vi "Serviceman.vi"() -> ()   [LabVIEW 2023]
uses:
  <vilib>/Utility/file.llb/Read Delimited Spreadsheet (string).vi
  <vilib>/Utility/file.llb/Write Delimited Spreadsheet (string).vi
panel:
  in  "Tab Control":T1(tab)=enum."Register_page"
  in  "register_btn":bool
  in  "login_btn":bool
  in  "password_login":string
  in  "username_login":string
  in  "home_btn":bool
  in  "back_to_login_btn":bool
  out "rgstr_status":string
  in  "email_address_rgstr":string
  in  "last_name_rgstr":string
  in  "first_name_rgstr":string
  in  "register_btn_rgstr":bool
  in  "password_rgstr":string
  in  "username_rgstr":string
  in  "logout_btn":bool
  # "Login"
  # "Username:"
  # "Password:"
  # "or Register"
  # "Registration"
  # "First Name:"
  # "Last Name:"
  # "Email Address:"
  # "Username:"
  # "Password:"
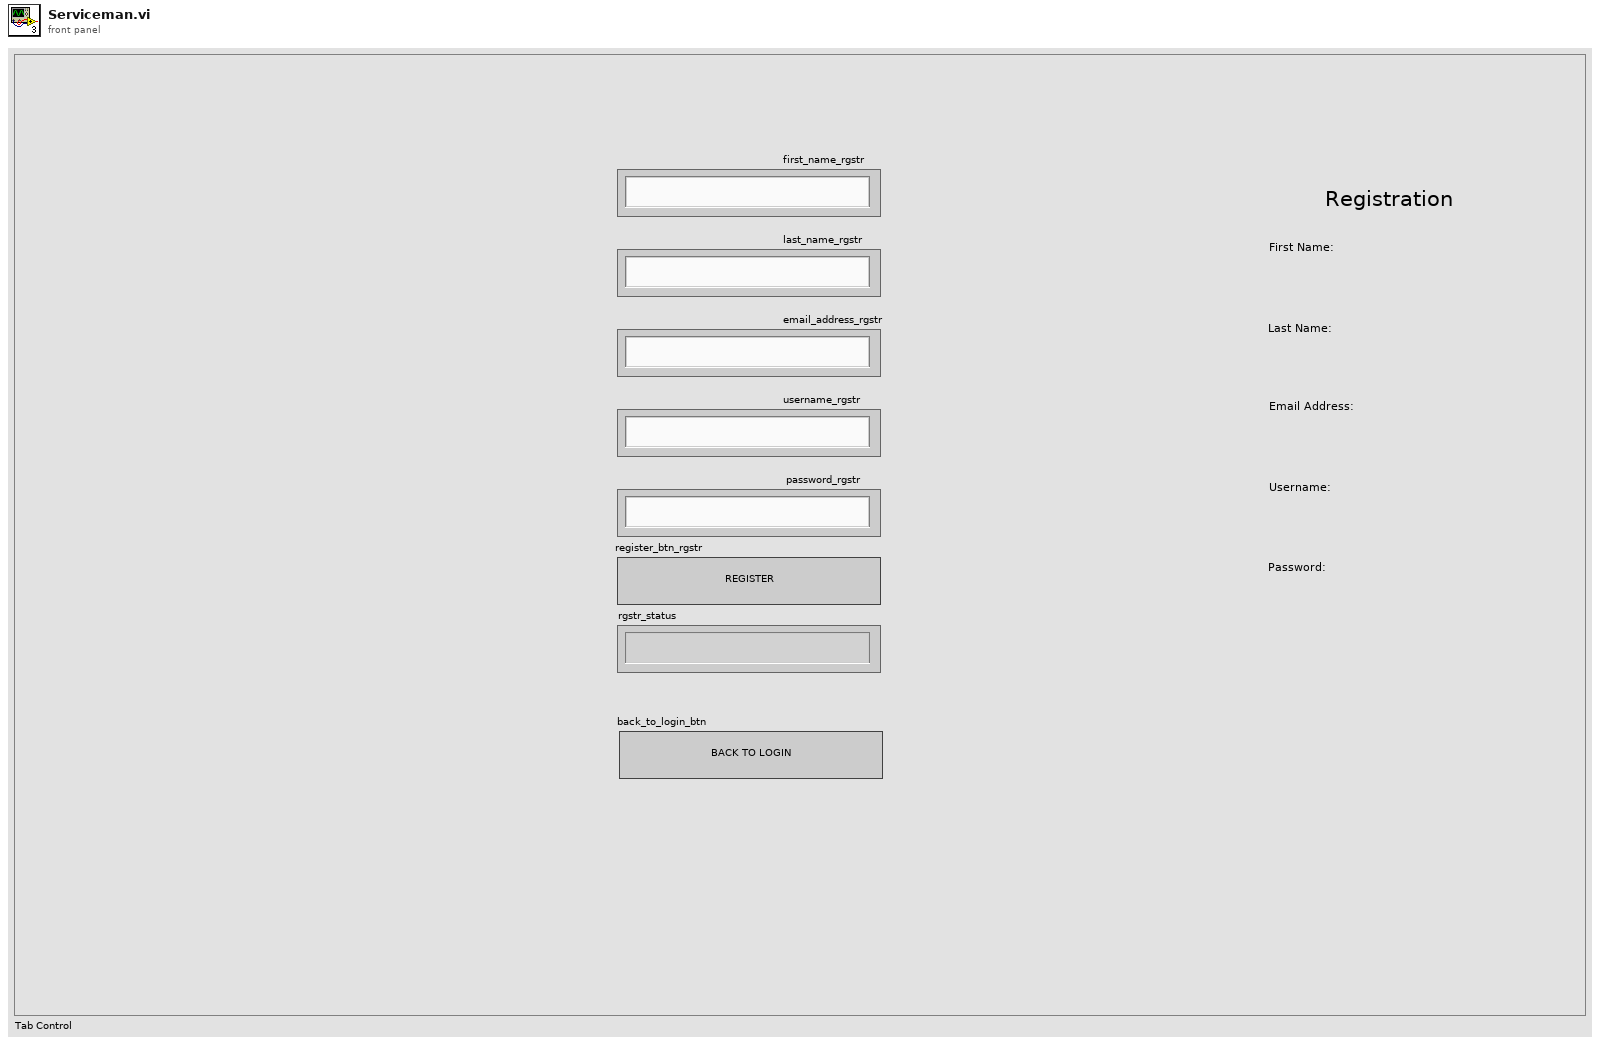
[diagram p1: front panel]
types:
  T1 = enum32{"Login_page", "Register_page", "Serviceman_page"}
  T2 = cluster{"Some":bool, "Tab Control":enum32{"Login_page", "Register_page", "Serviceman_page"}, "Probe":i32}
  T3 = enum16{"open", "replace", "create", "open or create", "replace or create", "replace or create with confirmation"}
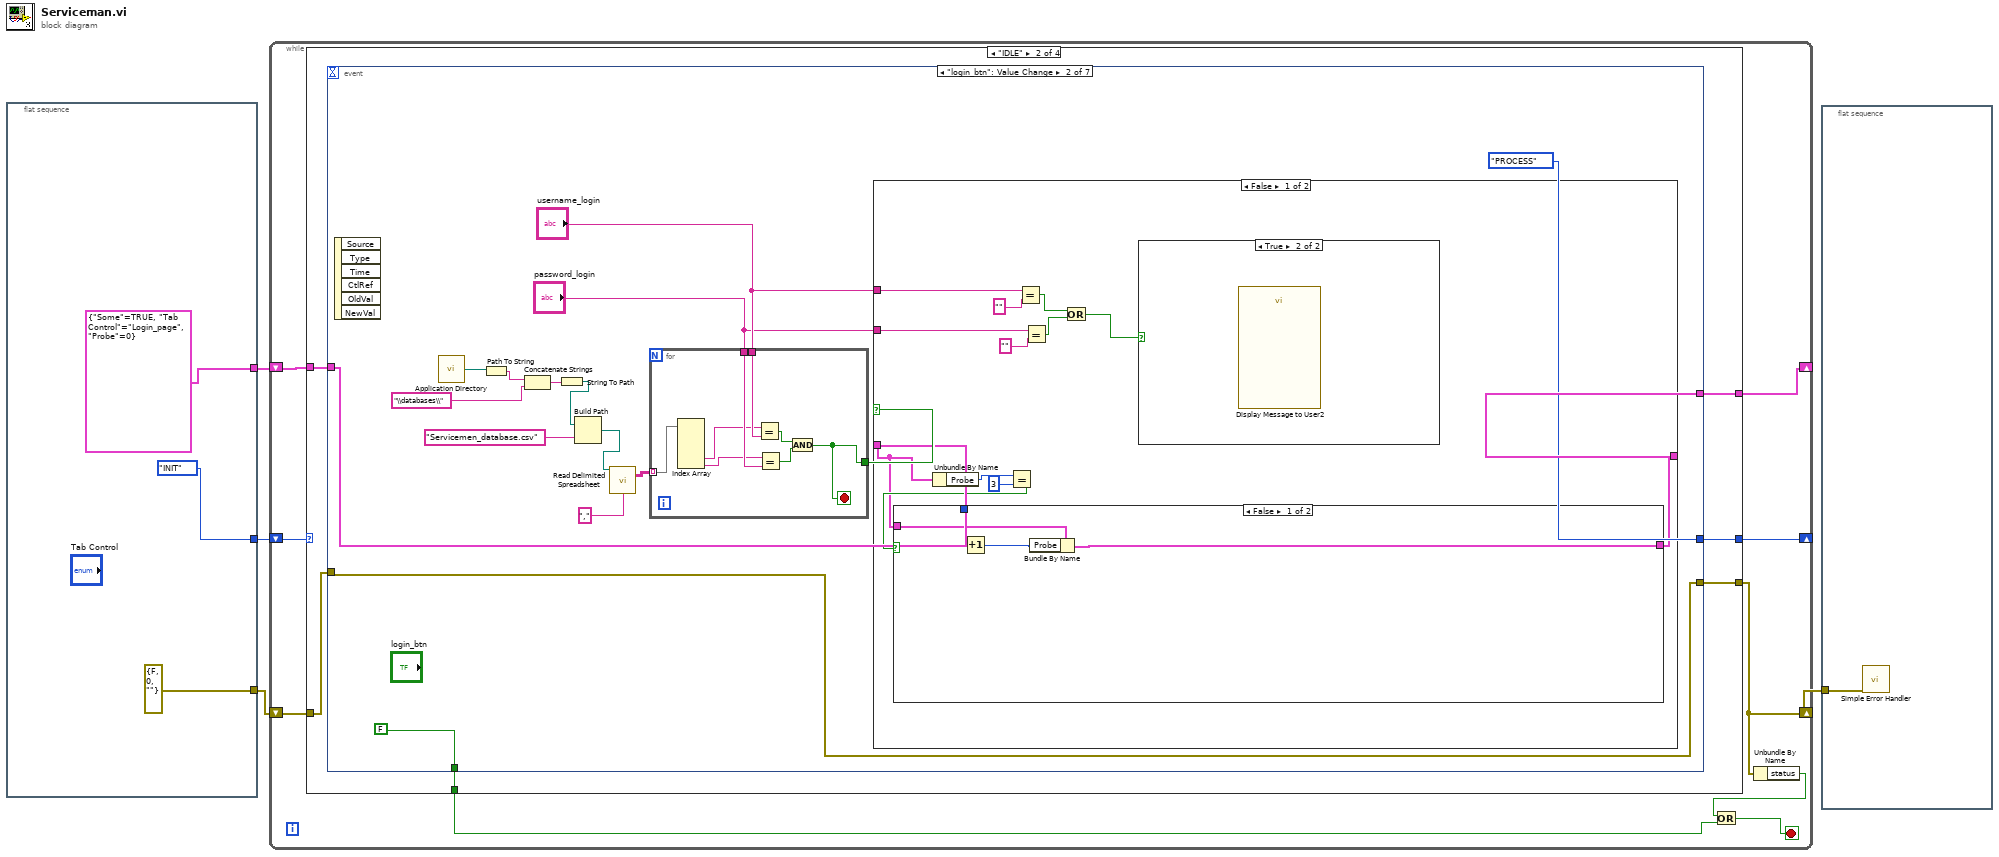
[diagram p0: block diagram]
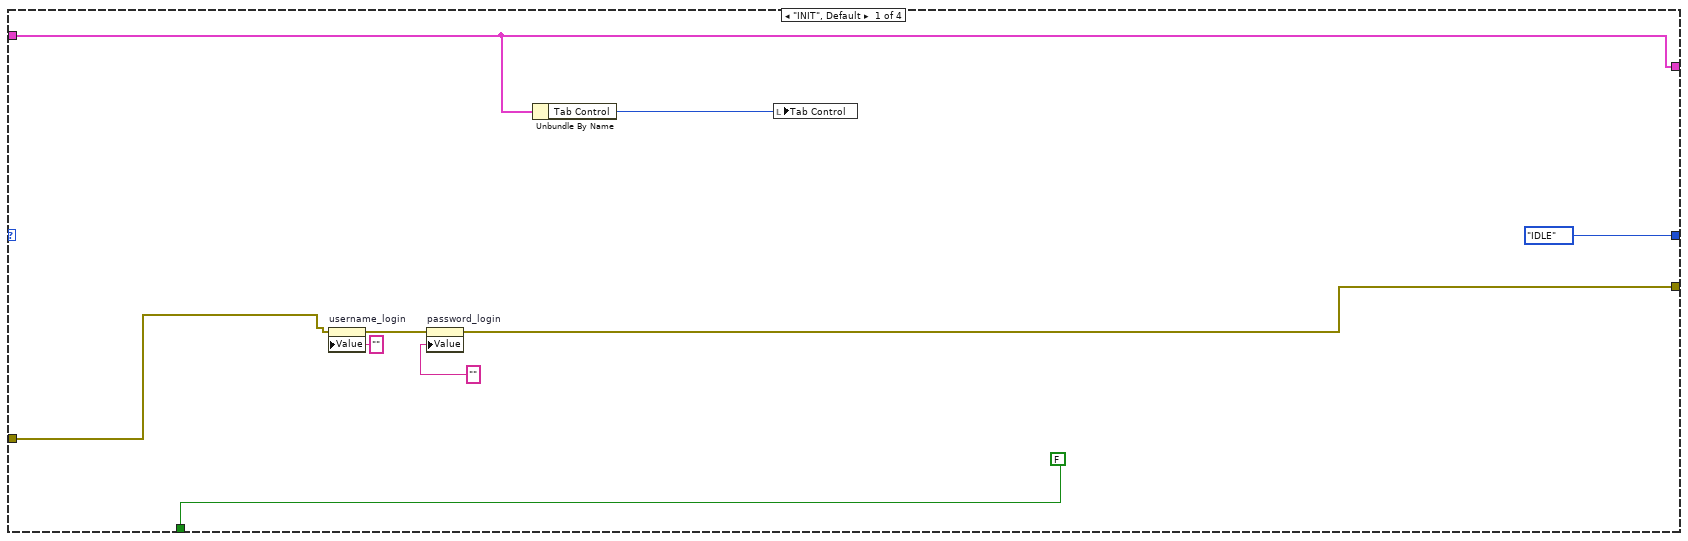
[diagram p2: hidden frame]
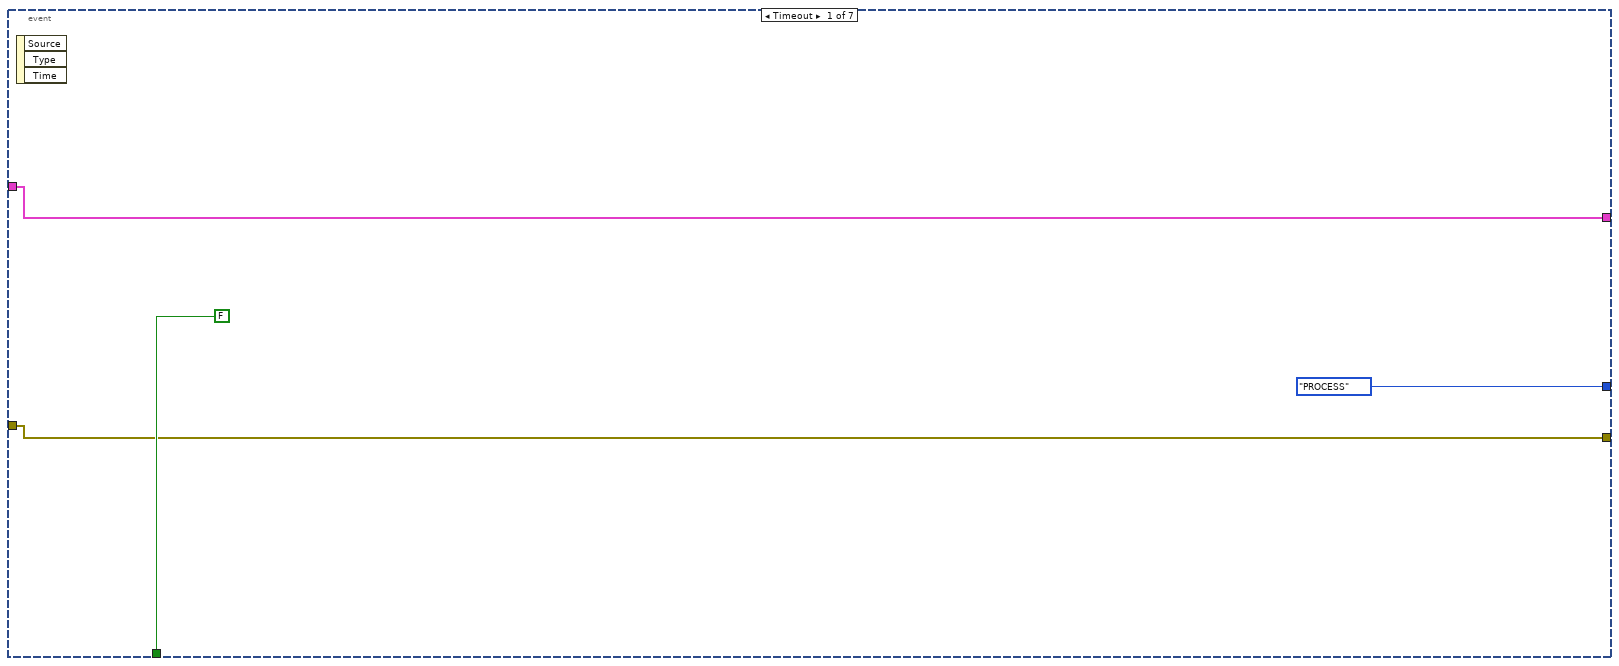
[diagram p3: hidden frame]
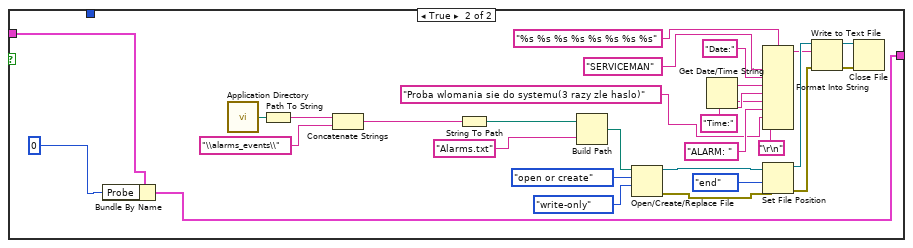
[diagram p4: hidden frame]
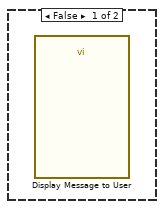
[diagram p5: hidden frame]
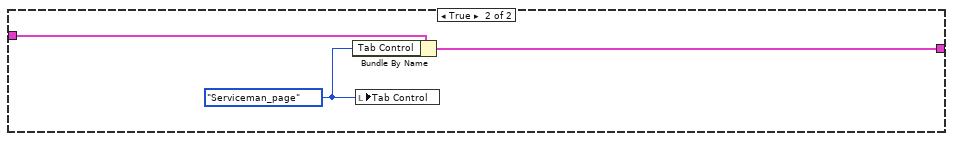
[diagram p6: hidden frame]
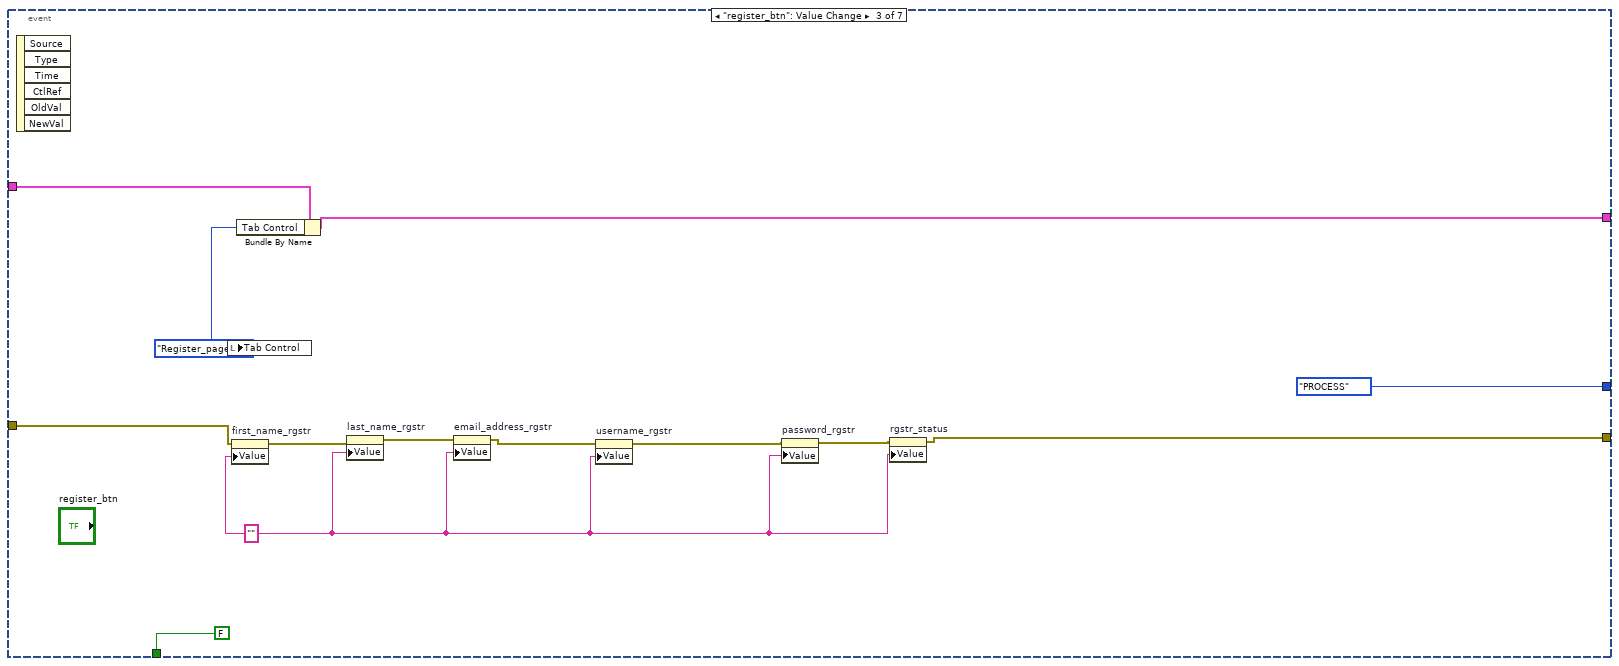
[diagram p7: hidden frame]
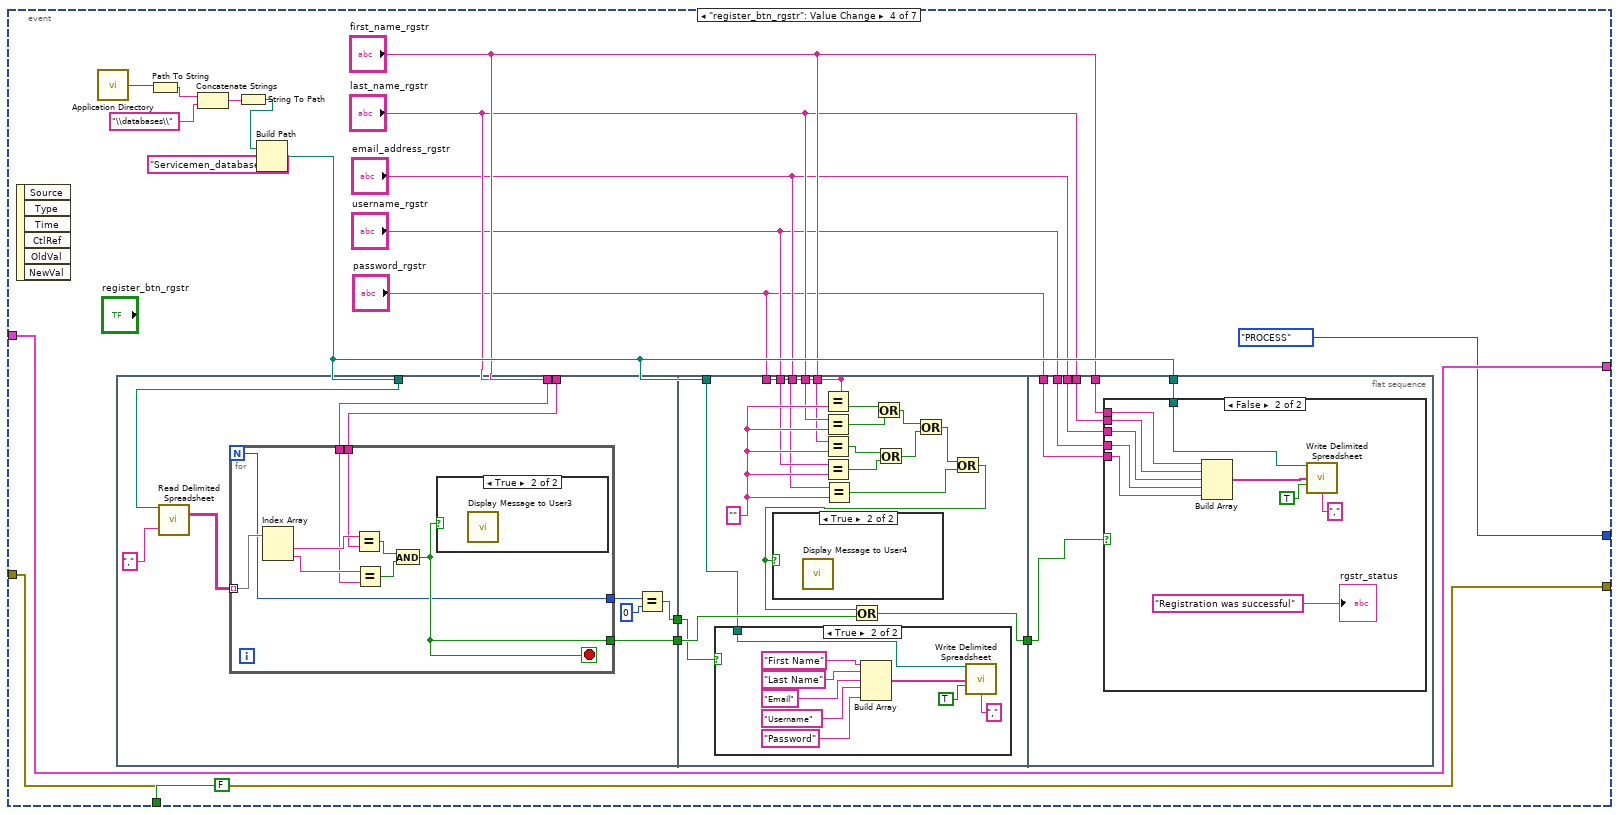
[diagram p8: hidden frame]
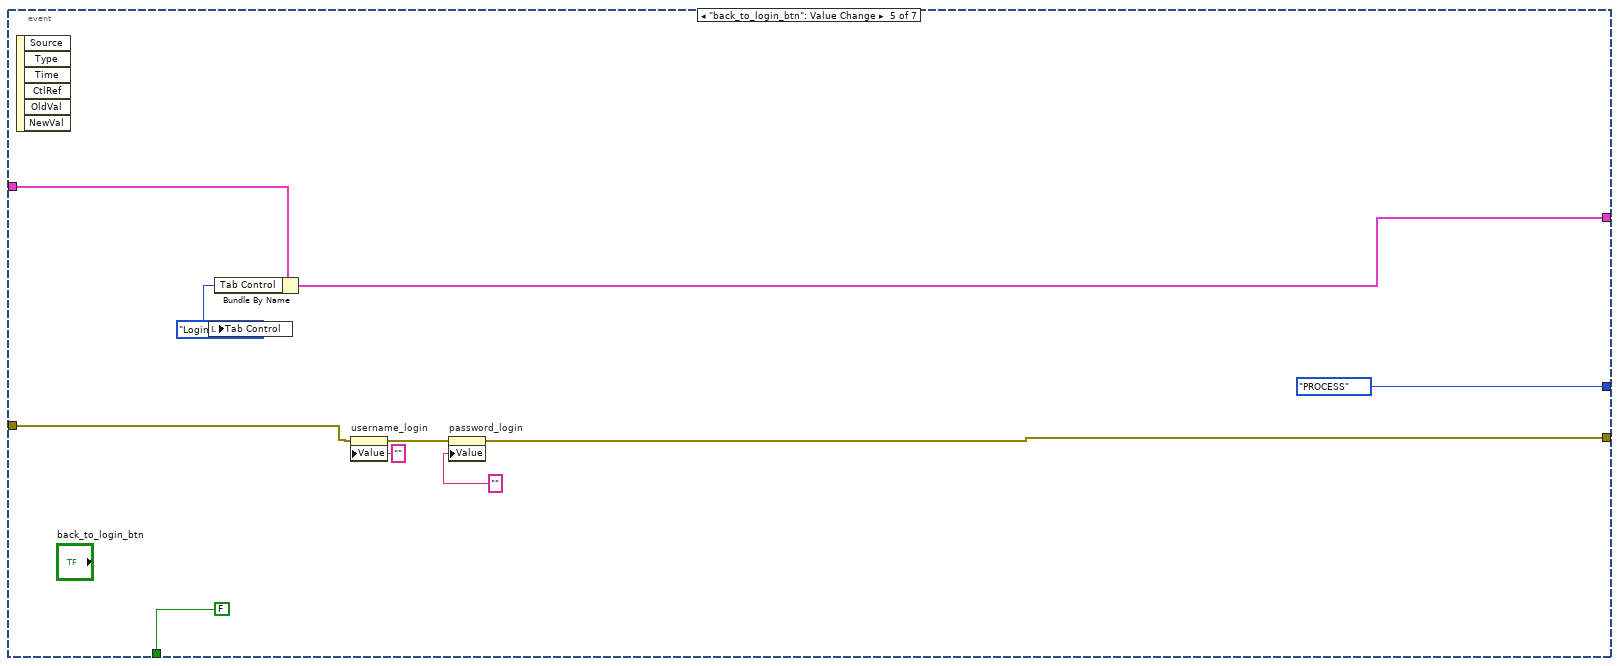
[diagram p13: hidden frame]
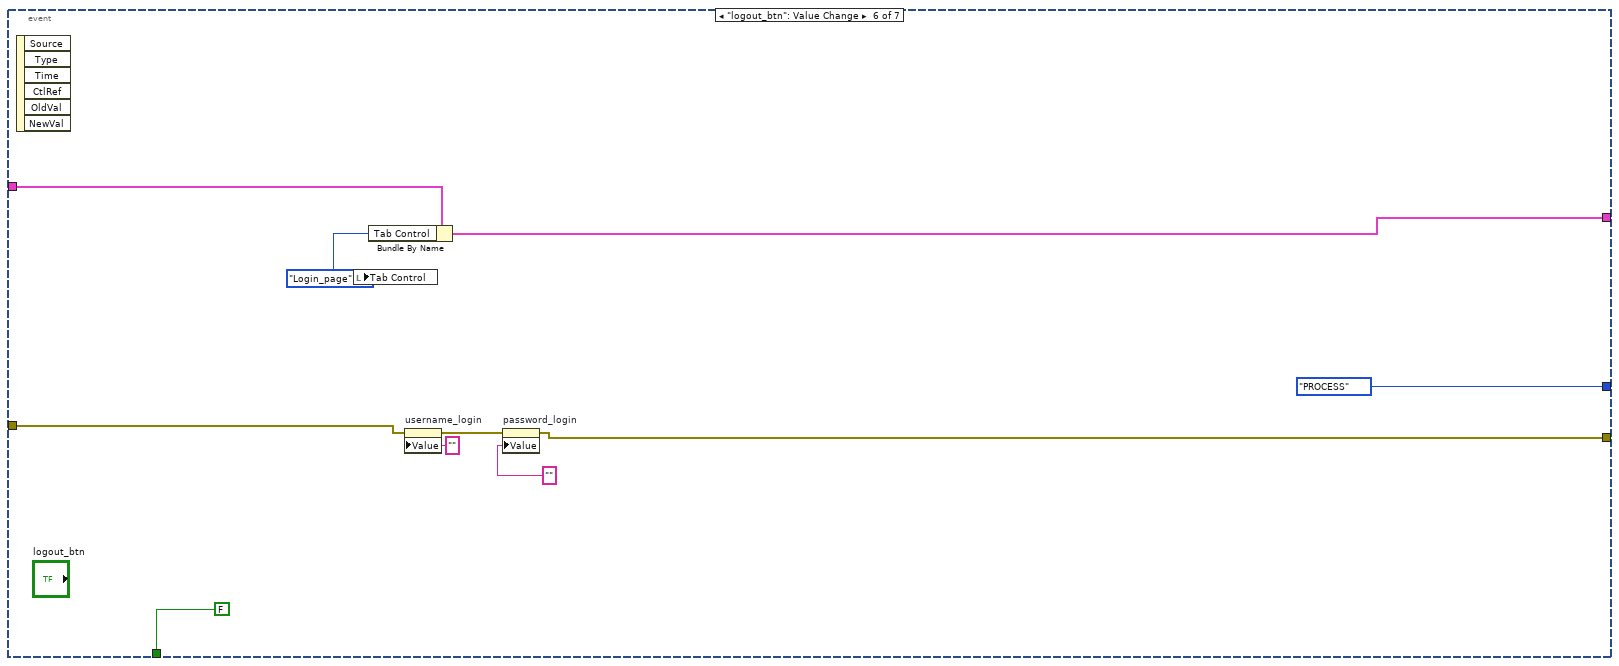
[diagram p14: hidden frame]
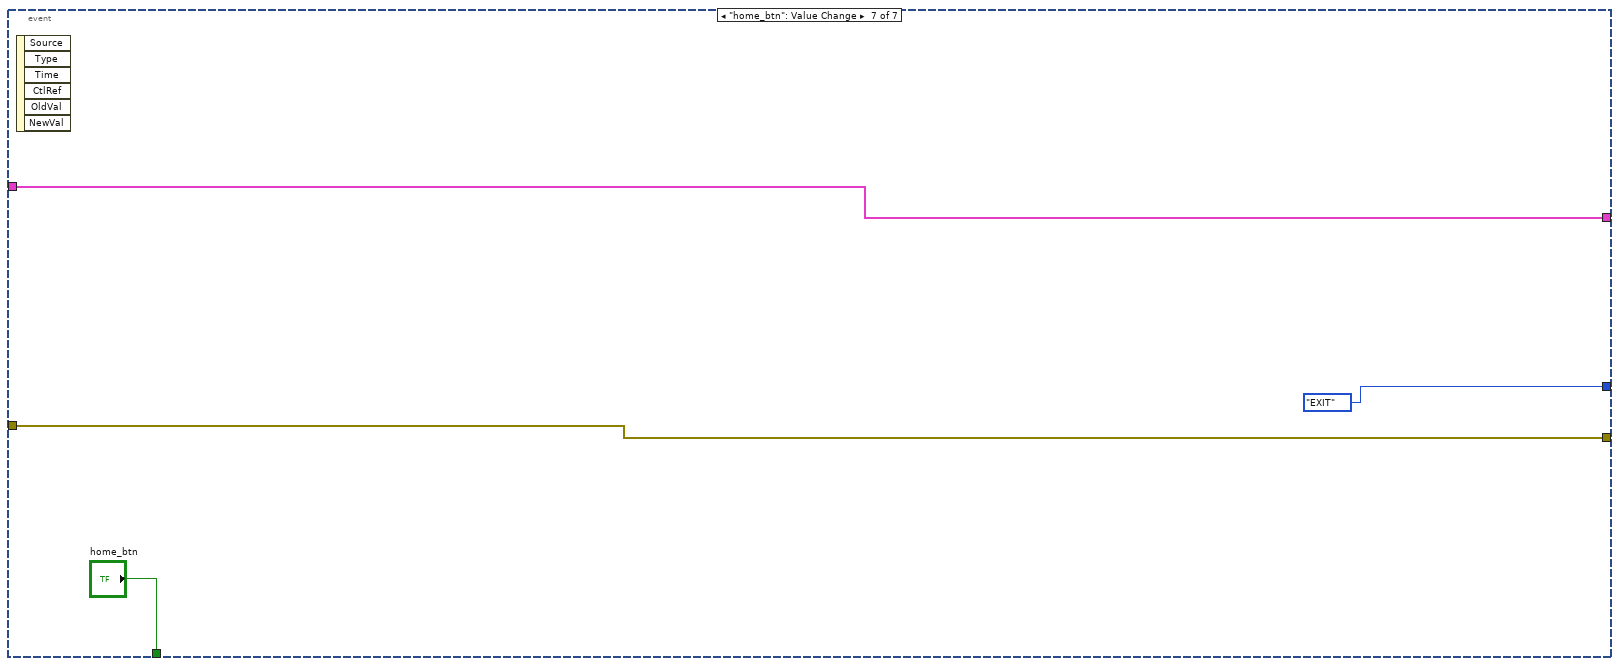
[diagram p15: hidden frame]
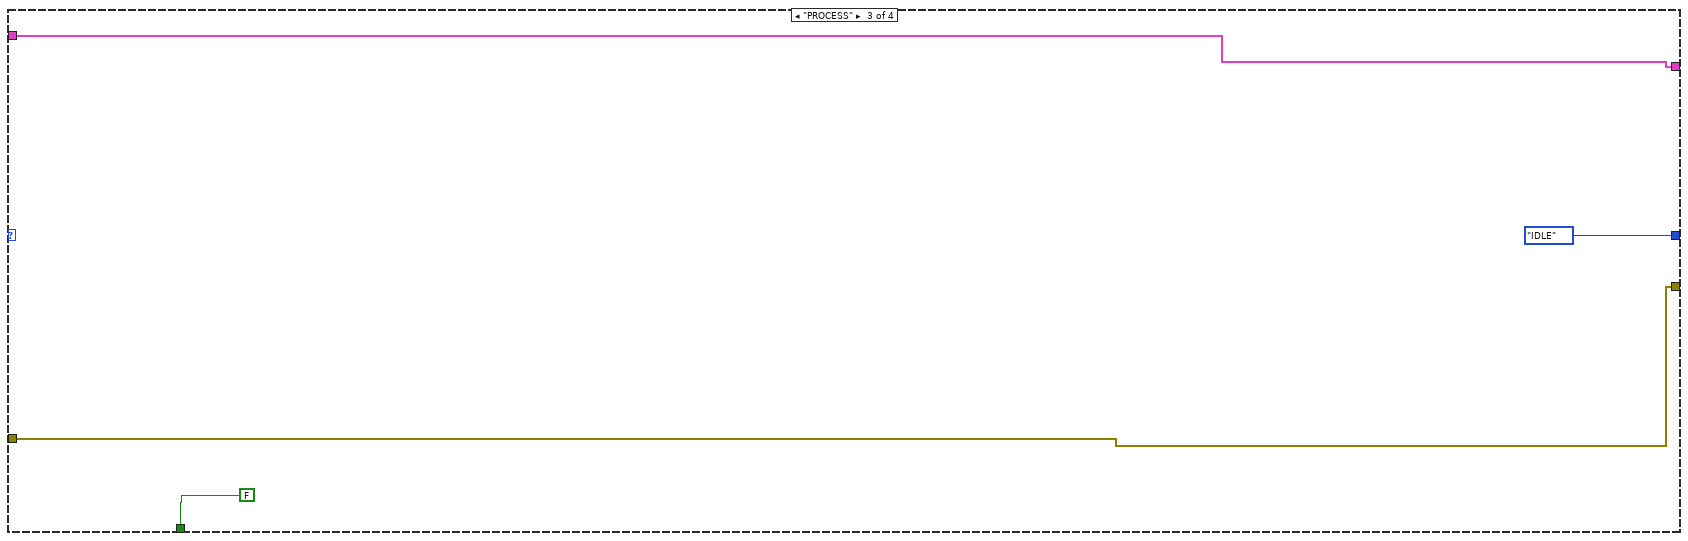
[diagram p16: hidden frame]
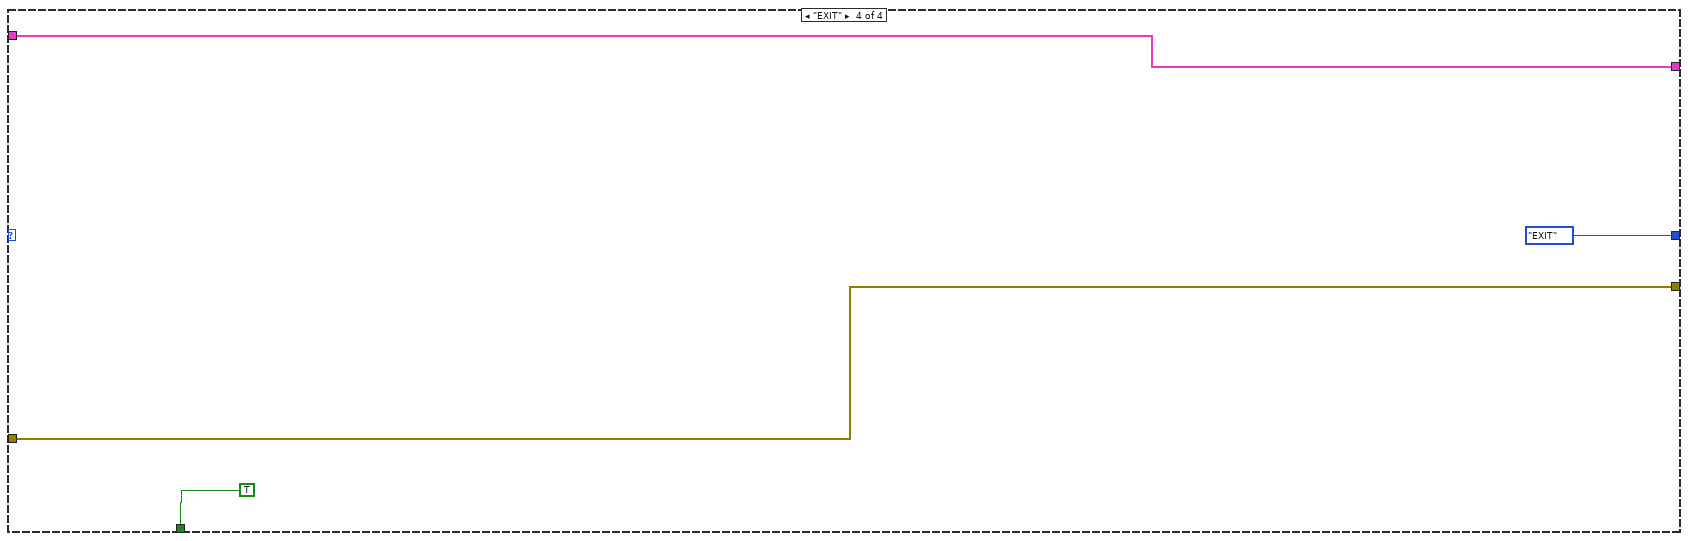
[diagram p17: hidden frame]
diagram:
  n1 = flat-sequence {
    tunnel: [enum16{"INIT", "IDLE", "PROCESS", "EXIT"}."INIT"] -> w4
    tunnel: [T2 {"Some"=TRUE, "Tab Control"=enum."Login_page", "Probe"=0}] -> w3
    tunnel: [errorcluster {"status"=FALSE, "code"=0, "source"=""} ("error constant")] -> w2
    frame #0 {
    }
  }
  n2 = while {
    shift-right: [w15] -> _
    shift-left: w4 -> [w16]
    shift-right: [w12] -> _
    shift-left: w3 -> [w13]
    shift-right: [w9] -> w1
    shift-left: w2 -> [w14]
    stop <- w10 stop-if-true
    n3 = case shown="\"IDLE\"" w16 {
      tunnel: [enum16{"INIT", "IDLE", "PROCESS", "EXIT"}."IDLE" w26 enum16{"INIT", "IDLE", "PROCESS", "EXIT"}."IDLE" enum16{"INIT", "IDLE", "PROCESS", "EXIT"}."EXIT"] -> w15
      tunnel: [FALSE ("stop") w27 FALSE ("stop") TRUE ("stop")] -> w11
      tunnel: w14 -> [w18 w31 w228 w233]
      tunnel: [w17 w30 w228 w233] -> w9
      tunnel: w13 -> [w22 w29 w229 w232]
      tunnel: [w22 w28 w229 w232] -> w12
      frame "INIT", Default {
        n4 = property on="username_login" class="Str"(error in=w18, "Value"="" ("username_login")) -> (error out=w21:errorcluster)  [unwired: 1 in, 1 out]
        n5 = property on="password_login" class="Str"(error in=w21, "Value"="" ("password_login")) -> (error out=w17:errorcluster)  [unwired: 1 in, 1 out]
        n6 = Unbundle By Name(w22) -> ("Tab Control"=w23:T1)
        n7 = local write "Tab Control"(w23) -> ()
      }
      frame "IDLE" {
        n8 = event shown="[1] \"login_btn\": Value Change" {
          selector: _ -> [_ _ _ _ _ _ _]
          dyn-events: _ -> [_ _ _ _ _ _ _]
          timeout: _ -> [_ _ _ _ _ _ _]
          tunnel: [FALSE ("stop") FALSE ("stop") FALSE ("home_btn") FALSE ("stop") FALSE ("stop") FALSE ("stop") "home_btn"] -> w27
          tunnel: w29 -> [w34 w46 w121 w139 w213 w223 w227]
          tunnel: [w34 w45 w120 w139 w212 w222 w227] -> w28
          tunnel: w31 -> [w33 w44 w114 w138 w206 w220 w226]
          tunnel: [w33 w44 w109 w138 w205 w217 w226] -> w30
          tunnel: [enum16{"INIT", "IDLE", "PROCESS", "EXIT"}."PROCESS" enum16{"INIT", "IDLE", "PROCESS", "EXIT"}."PROCESS" enum16{"INIT", "IDLE", "PROCESS", "EXIT"}."PROCESS" enum16{"INIT", "IDLE", "PROCESS", "EXIT"}."PROCESS" enum16{"INIT", "IDLE", "PROCESS", "EXIT"}."PROCESS" enum16{"INIT", "IDLE", "PROCESS", "EXIT"}."PROCESS" enum16{"INIT", "IDLE", "PROCESS", "EXIT"}."EXIT"] -> w26
          event Timeout {
            n9 = event-data() -> ()  [unwired: 1 in, 3 out]
          }
          event "login_btn": Value Change {
            n10 = event-data() -> ()  [unwired: 1 in, 6 out]
            n11 = call <vilib>:"Application Directory.vi"() -> ("Application Directory"=w40:path)
            n12 = Path To String(path=w40) -> (string=w39:string)
            n13 = Concatenate Strings(w39, "\\databases\\") -> (w37:string)
            n14 = String To Path(string=w37) -> (path=w36:path)
            n15 = Build Path(base path=w36, name or relative path="Servicemen_database.csv") -> (appended path=w50:path)
            n16 = call-poly <vilib>:"Read Delimited Spreadsheet.vi"("file path (dialog if empty)"=w50, "delimiter (\\t)"="," ("delimiter (\\t)")) -> ("all rows"=w48:string[][])  [unwired: 8 in, 5 out]
            n17 = for {
              tunnel: w48 -> [w108] mode=indexing
              tunnel: "username_login" -> [w107]
              tunnel: "password_login" -> [w106]
              tunnel: [w103] -> w47
              stop <- w103 stop-if-true
              n18 = Index Array(array=w108) -> (element #4=w101:string, element #5=w102:string)  [unwired: 5 in, 3 out]
              n19 = Equal?(x=w101, y=w107) -> (x = y?=w105:bool)
              n20 = Equal?(x=w102, y=w106) -> (x = y?=w104:bool)
              n21 = And(x=w105, y=w104) -> (x .and. y?=w103:bool)
            }
            n22 = case shown="False" w47 {
              tunnel: w46 -> [w55 w100]
              tunnel: [w54 w99] -> w45
              tunnel: "username_login" -> [w64 _]
              tunnel: "password_login" -> [w61 _]
              frame False {
                n23 = Unbundle By Name(w55) -> ("Probe"=w53:i32)
                n24 = Equal?(x=w53, y=3) -> (x = y?=w56:bool)
                n25 = case shown="False" w56 {
                  tunnel: [w67 w70] -> w54
                  tunnel: w55 -> [w68 w71]
                  tunnel: w53 -> [w65 _]
                  frame False {
                    n26 = Increment(x=w65) -> (x+1=w66:i32)
                    n27 = Bundle By Name(cluster=w68, "Probe"=w66) -> (w67:T2)
                  }
                  frame True {
                    n28 = Bundle By Name(cluster=w71, "Probe"=0) -> (w70:T2)
                    n29 = call <vilib>:"Application Directory.vi"() -> ("Application Directory"=w78:path)
                    n30 = Path To String(path=w78) -> (string=w77:string)
                    n31 = Concatenate Strings(w77, "\\alarms_events\\") -> (w75:string)
                    n32 = String To Path(string=w75) -> (path=w74:path)
                    n33 = Build Path(base path=w74, name or relative path="Alarms.txt") -> (appended path=w73:path)
                    n34 = Open/Create/Replace File(file path (use dialog)=w73, operation (0:open)=T3."open or create", access (0:read/write)=enum16{"read/write", "read-only", "write-only"}."write-only") -> (refnum out=w96:refnum<file>, error out=w97:errorcluster)  [unwired: 3 in, 1 out]
                    n35 = Get Date/Time String() -> (date string=w85:string, time string=w83:string)  [unwired: 3 in]
                    n36 = Format Into String(format string="%s %s %s %s %s %s %s %s", "SERVICEMAN" ("format string"), "Date:" ("format string"), w85, "Time:" ("format string"), w83, "ALARM: " ("format string"), "Proba wlomania sie do systemu(3 razy zle haslo)" ("format string"), "\r\n") -> (resulting string=w80:string)  [unwired: 2 in, 1 out]
                    n37 = Set File Position(refnum=w96, from (0:start)=enum16{"start", "end", "current"}."end", error in=w97) -> (refnum out=w93:refnum<file>, error out=w92:errorcluster)  [unwired: 1 in]
                    n38 = Write to Text File(file (use dialog)=w93, text=w80, error in=w92) -> (refnum out=w94:refnum<file>, error out=w95:errorcluster)  [unwired: 1 in, 1 out]
                    n39 = Close File(refnum=w94, error in=w95) -> ()  [unwired: 2 out]
                  }
                }
                n40 = Equal?(x=w64, y="") -> (x = y?=w60:bool)
                n41 = Equal?(x=w61, y="") -> (x = y?=w59:bool)
                n42 = Or(x=w60, y=w59) -> (x .or. y?=w58:bool)
                n43 = case shown="True" w58 {
                  frame False {
                    n44 = call "Display Message to User"() -> ()  [unwired: 10 in, 2 out]
                  }
                  frame True {
                    n45 = call "Display Message to User2"() -> ()  [unwired: 10 in, 2 out]
                  }
                }
              }
              frame True {
                w98 = T1."Serviceman_page" ("Tab Control")
                n46 = Bundle By Name(cluster=w100, "Tab Control"=w98) -> (w99:T2)
                n47 = local write "Tab Control"(w98) -> ()
              }
            }
          }
          event "register_btn": Value Change {
            w119 = T1."Register_page" ("Tab Control")
            w111 = ""
            n48 = event-data() -> ()  [unwired: 1 in, 6 out]
            n49 = local write "Tab Control"(w119) -> ()
            n50 = property on="first_name_rgstr" class="Str"(error in=w114, "Value"=w111) -> (error out=w118:errorcluster)  [unwired: 1 in, 1 out]
            n51 = Bundle By Name(cluster=w121, "Tab Control"=w119) -> (w120:T2)
            n52 = property on="last_name_rgstr" class="Str"(error in=w118, "Value"=w111) -> (error out=w117:errorcluster)  [unwired: 1 in, 1 out]
            n53 = property on="email_address_rgstr" class="Str"(error in=w117, "Value"=w111) -> (error out=w116:errorcluster)  [unwired: 1 in, 1 out]
            n54 = property on="username_rgstr" class="Str"(error in=w116, "Value"=w111) -> (error out=w115:errorcluster)  [unwired: 1 in, 1 out]
            n55 = property on="password_rgstr" class="Str"(error in=w115, "Value"=w111) -> (error out=w110:errorcluster)  [unwired: 1 in, 1 out]
            n56 = property on="rgstr_status" class="Str"(error in=w110, "Value"=w111) -> (error out=w109:errorcluster)  [unwired: 1 in, 1 out]
          }
          event "register_btn_rgstr": Value Change {
            n57 = event-data() -> ()  [unwired: 1 in, 6 out]
            n58 = call <vilib>:"Application Directory.vi"() -> ("Application Directory"=w135:path)
            n59 = flat-sequence {
              tunnel: "first_name_rgstr" -> [w145]
              tunnel: "last_name_rgstr" -> [w144]
              tunnel: [w147] -> w130
              tunnel: w127 -> [w146]
              tunnel: [w142] -> w129
              tunnel: w130 -> [w165]
              tunnel: [w164] -> w128
              tunnel: [w161] -> _
              tunnel: "last_name_rgstr" -> [w168]
              tunnel: [w160] -> _
              tunnel: "username_rgstr" -> [w167]
              tunnel: [w159] -> _
              tunnel: w129 -> [w163]
              tunnel: w127 -> [w162]
              tunnel: "first_name_rgstr" -> [w161]
              tunnel: "email_address_rgstr" -> [w160]
              tunnel: "password_rgstr" -> [w159]
              tunnel: w128 -> [w187]
              tunnel: w127 -> [w193]
              tunnel: "first_name_rgstr" -> [w192]
              tunnel: "last_name_rgstr" -> [w191]
              tunnel: "email_address_rgstr" -> [w190]
              tunnel: "username_rgstr" -> [w189]
              tunnel: "password_rgstr" -> [w188]
              frame #0 {
                n60 = call-poly <vilib>:"Read Delimited Spreadsheet.vi"("file path (dialog if empty)"=w146, "delimiter (\\t)"="," ("delimiter (\\t)")) -> ("all rows"=w148:string[][])  [unwired: 8 in, 5 out]
                n61 = for {
                  N -> [w150]
                  tunnel: w148 -> [w152] mode=indexing
                  tunnel: w145 -> [w156]
                  tunnel: w144 -> [w155]
                  tunnel: [w151] -> w147
                  tunnel: [w150] -> w141
                  stop <- w151 stop-if-true
                  n62 = Index Array(array=w152) -> (element #1=w158:string, element #2=w157:string)  [unwired: 2 in]
                  n63 = Equal?(x=w158, y=w156) -> (x = y?=w154:bool)
                  n64 = Equal?(x=w157, y=w155) -> (x = y?=w153:bool)
                  n65 = And(x=w154, y=w153) -> (x .and. y?=w151:bool)
                  n66 = case shown="True" w151 {
                    frame False {
                    }
                    frame True {
                      n67 = call "Display Message to User3"() -> ()  [unwired: 10 in, 2 out]
                    }
                  }
                }
                n68 = Equal?(x=w141, y=0) -> (x = y?=w142:bool)
              }
              frame #1 {
                w169 = "" ("delimiter (\\t)")
                n69 = case shown="True" w163 {
                  tunnel: w162 -> [_ w178]
                  frame False {
                  }
                  frame True {
                    n70 = Build Array("First Name", "Last Name", "Email", "Username", "Password") -> (w183:string[])
                    n71 = call-poly <vilib>:"Write Delimited Spreadsheet.vi"("file path (dialog if empty)"=w178, "1D data"=w183, "append to file? (new file:F)"=TRUE, "delimiter (\\t)"="," ("delimiter (\\t)")) -> ()  [unwired: 10 in, 2 out]
                  }
                }
                n72 = Equal?(x=w161, y=w169) -> (x = y?=w177:bool)
                n73 = Equal?(x=w168, y=w169) -> (x = y?=w176:bool)
                n74 = Equal?(x=w160, y=w169) -> (x = y?=w175:bool)
                n75 = Equal?(x=w167, y=w169) -> (x = y?=w174:bool)
                n76 = Equal?(x=w159, y=w169) -> (x = y?=w170:bool)
                n77 = Or(x=w177, y=w176) -> (x .or. y?=w173:bool)
                n78 = Or(x=w175, y=w174) -> (x .or. y?=w172:bool)
                n79 = Or(x=w173, y=w172) -> (x .or. y?=w171:bool)
                n80 = Or(x=w171, y=w170) -> (x .or. y?=w166:bool)
                n81 = case shown="True" w166 {
                  frame False {
                  }
                  frame True {
                    n82 = call "Display Message to User4"() -> ()  [unwired: 10 in, 2 out]
                  }
                }
                n83 = Or(x=w166, y=w165) -> (x .or. y?=w164:bool)
              }
              frame #2 {
                n84 = case shown="False" w187 {
                  tunnel: w193 -> [_ w200]
                  tunnel: w192 -> [_ w199]
                  tunnel: w191 -> [_ w198]
                  tunnel: w190 -> [_ w197]
                  tunnel: w189 -> [_ w196]
                  tunnel: w188 -> [_ w195]
                  frame True {
                  }
                  frame False {
                    n85 = Build Array(w199, w198, w197, w196, w195) -> (w203:string[])
                    n86 = call-poly <vilib>:"Write Delimited Spreadsheet.vi"("file path (dialog if empty)"=w200, "1D data"=w203, "append to file? (new file:F)"=TRUE, "delimiter (\\t)"="," ("delimiter (\\t)")) -> ()  [unwired: 10 in, 2 out]
                    "rgstr_status" <- "Registration was successful" ("rgstr_status")
                  }
                }
              }
            }
            n87 = Path To String(path=w135) -> (string=w134:string)
            n88 = Concatenate Strings(w134, "\\databases\\") -> (w132:string)
            n89 = String To Path(string=w132) -> (path=w131:path)
            n90 = Build Path(base path=w131, name or relative path="Servicemen_database.csv") -> (appended path=w127:path)
          }
          event "back_to_login_btn": Value Change {
            w207 = T1."Login_page" ("Tab Control")
            n91 = event-data() -> ()  [unwired: 1 in, 6 out]
            n92 = local write "Tab Control"(w207) -> ()
            n93 = Bundle By Name(cluster=w213, "Tab Control"=w207) -> (w212:T2)
            n94 = property on="username_login" class="Str"(error in=w206, "Value"="" ("username_login")) -> (error out=w209:errorcluster)  [unwired: 1 in, 1 out]
            n95 = property on="password_login" class="Str"(error in=w209, "Value"="" ("password_login")) -> (error out=w205:errorcluster)  [unwired: 1 in, 1 out]
          }
          event "logout_btn": Value Change {
            w221 = T1."Login_page" ("Tab Control")
            n96 = event-data() -> ()  [unwired: 1 in, 6 out]
            n97 = local write "Tab Control"(w221) -> ()
            n98 = Bundle By Name(cluster=w223, "Tab Control"=w221) -> (w222:T2)
            n99 = property on="username_login" class="Str"(error in=w220, "Value"="" ("username_login")) -> (error out=w218:errorcluster)  [unwired: 1 in, 1 out]
            n100 = property on="password_login" class="Str"(error in=w218, "Value"="" ("password_login")) -> (error out=w217:errorcluster)  [unwired: 1 in, 1 out]
          }
          event "home_btn": Value Change {
            n101 = event-data() -> ()  [unwired: 1 in, 6 out]
          }
        }
      }
      frame "PROCESS" {
      }
      frame "EXIT" {
      }
    }
    n102 = Unbundle By Name(w9) -> ("status"=w8:bool)
    n103 = Or(x=w8, y=w11) -> (x .or. y?=w10:bool)
  }
  n104 = flat-sequence {
    tunnel: w1 -> [w236]
    frame #0 {
      n105 = call <vilib>:"Simple Error Handler.vi"("error in (no error)"=w236) -> ()  [unwired: 4 in, 5 out]
    }
  }
